vi "Write OPC UA.vi"() -> ()   [LabVIEW 2018]
uses:
  <vilib>/OPCUA/controls/NodeId.ctl
  <vilib>/OPCUA/controls/Write Status.ctl
  <vilib>/OPCUA/client/Multiple Write Double.vi
  <vilib>/OPCUA/NI OPC UA Client.lvlib
panel:
  out "Temperature Value":dbl
  in  "Node Id":string
  in  "Server Endpoint URL":string
  in  "stop":bool
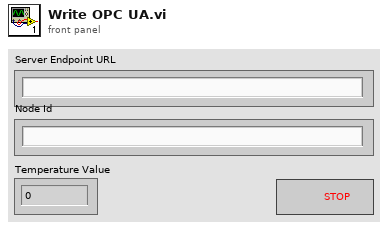
[diagram p1: front panel]
types:
  T1 = cluster{"message mode":enum16{"None", "Sign", "Sign and Encrypt"}, "security":enum16{"Basic256", "Basic128Rsa15"}}
  T2 = typedef "OPC UA Client Refnum.ctl" = refnum<k21>
  T3 = typedef "NodeId.ctl" = string
  T4 = typedef "Write Status.ctl" = u32
  T5 = cluster{"node ID":T3, "value":dbl, "timestamp (current time)":timestamp, "node status":T4}
  T6 = cluster{"node ID":T3, "value":dbl, "timestamp (current time)":timestamp, "node status":T4}[]
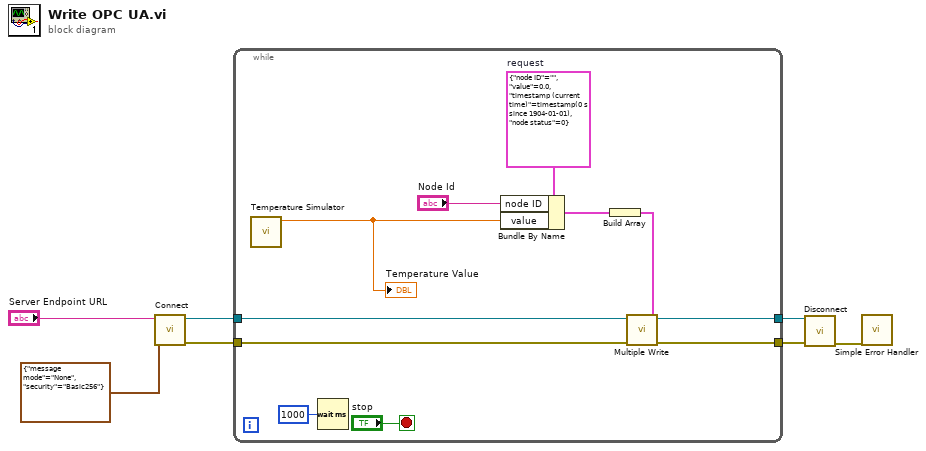
[diagram p0: block diagram]
diagram:
  n1 = call <vilib>:"Connect.vi"("security policy"=T1 {"message mode"=enum."None", "security"=enum."Basic256"}, "server endpoint URL"="Server Endpoint URL") -> ("error out"=w4:errorcluster, "OPC UA client refnum out"=w5:T2)  [unwired: 7 in, 1 out]
  n2 = while {
    tunnel: w5 -> [w16]
    tunnel: w4 -> [w15]
    tunnel: [w9] -> w2
    tunnel: [w8] -> w3
    stop <- "stop" stop-if-true
    w11 = T5 {"node ID"="", "value"=0.0, "timestamp (current time)"=timestamp(0 s since 1904-01-01), "node status"=0}  # request
    n3 = call "Temperature Simulator.vi"() -> ("Temperature Value"=w14:dbl)  [unwired: 11 in]
    "Temperature Value" <- w14
    n4 = Wait (ms)(milliseconds to wait=u32 1000) -> ()  [unwired: 1 out]
    n5 = Bundle By Name "Bundle By Name"(cluster=w11, "node ID"="Node Id", "value"=w14) -> (w12:T5)
    n6 = Build Array(w12) -> (w10:T6)
    n7 = call-poly <vilib>:"Multiple Write.vi"("error in (no error)"=w15, "requests"=w10, "OPC UA client refnum in"=w16) -> ("error out"=w9:errorcluster, "OPC UA client refnum out"=w8:T2)  [unwired: 5 in, 2 out]
  }
  n8 = call <vilib>:"Disconnect.vi"("error in (no error)"=w2, "OPC UA client refnum in"=w3) -> ("error out"=w1:errorcluster)  [unwired: 9 in]
  n9 = call <vilib>:"Simple Error Handler.vi"("error in (no error)"=w1) -> ()  [unwired: 4 in, 5 out]
